vi "Value Pair Page.vi"() -> ()   [LabVIEW 2020, in "3D Plot.lvclass"]
uses:
  <vilib>/Math Plots/3D Math Plots/3D Plot/3D Plot/3D Plot.lvclass
  <vilib>/Math Plots/3D Math Plots/3D Plot/3D Plot/Typedef/Value Pair Property.ctl
  <vilib>/Math Plots/3D Math Plots/3D Plot/3D Plot/Typedef/Value Pair Cluster.ctl
  <vilib>/Math Plots/3D Math Plots/3D Plot/3D Plot/Typedef/Dialog State.ctl
  <vilib>/Math Plots/3D Math Plots/3D Plot/3D Plot/Typedef/Temp Scene State.ctl
  <vilib>/Math Plots/3D Math Plots/3D Plot/3D Plot/Typedef/Temp Scene Property Action.ctl
panel:
  in  "Move Down":bool caption="Move down"
  in  "Move Up":bool caption="Move up"
  in  "Delete":bool
  in  "New":bool
  in  "Active Axis":u16(ring) caption="Active axis" items=["X Axis", "Y Axis", "Z Axis"]
  in  "Label Mode":u16(ring) caption="Label mode" items=["Name", "Value", "None "]
  in  "Show Tick":bool caption="Show tick"
  in  "Show Grid":bool caption="Show grid"
  in  "Value":sgl
  in  "Name":string
  in  "Value Pair List":i32(listbox) caption="Value pair list"
  out "Value Pair Property Out":T1
  in  "Value Pair Property In":T1
  in  "Event Registration":refnum<event-registration>
  # "Value Pair"
  # "Display Style"
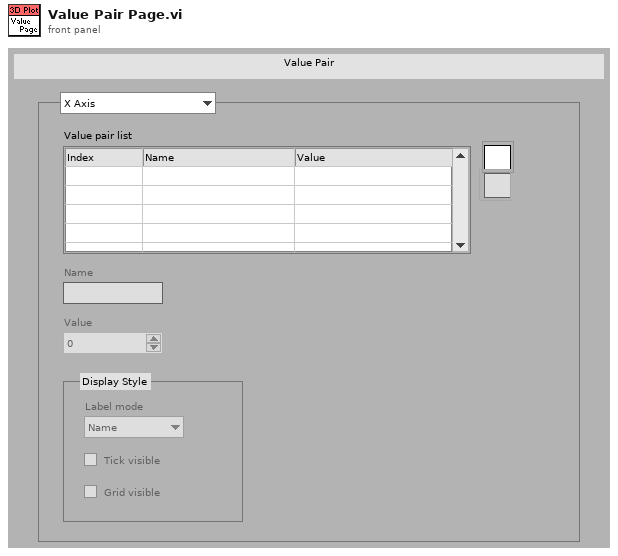
[diagram p1: front panel]
types:
  T1 = typedef "3D Plot.lvclass/Value Pair Property.ctl" = T2[]
  T2 = typedef "3D Plot.lvclass/Value Pair Cluster.ctl" = cluster{"Value Pair Array":cluster{"Value":sgl, "Name":string}[], "Show Tick":bool, "Show Grid":bool, " Label Mode":enum16{"Name", "Value", "None"}}
  T3 = typedef "3D Plot.lvclass/Dialog State.ctl" = enum16{"Initialize", "Read Porperty", "Write Property", "Idle", "Exit"}
  T4 = typedef "3D Plot.lvclass/Temp Scene Property Action.ctl" = enum16{"Graph Property", "Light Property", "Axis Property", "Value Pair Property", "Format Property", "Cursor Property", "Plot Specific Property"}
  T5 = typedef "3D Plot.lvclass/Temp Scene State.ctl" = enum16{"Create", "Update Scene", "Get Plot Representation", "Destory"}
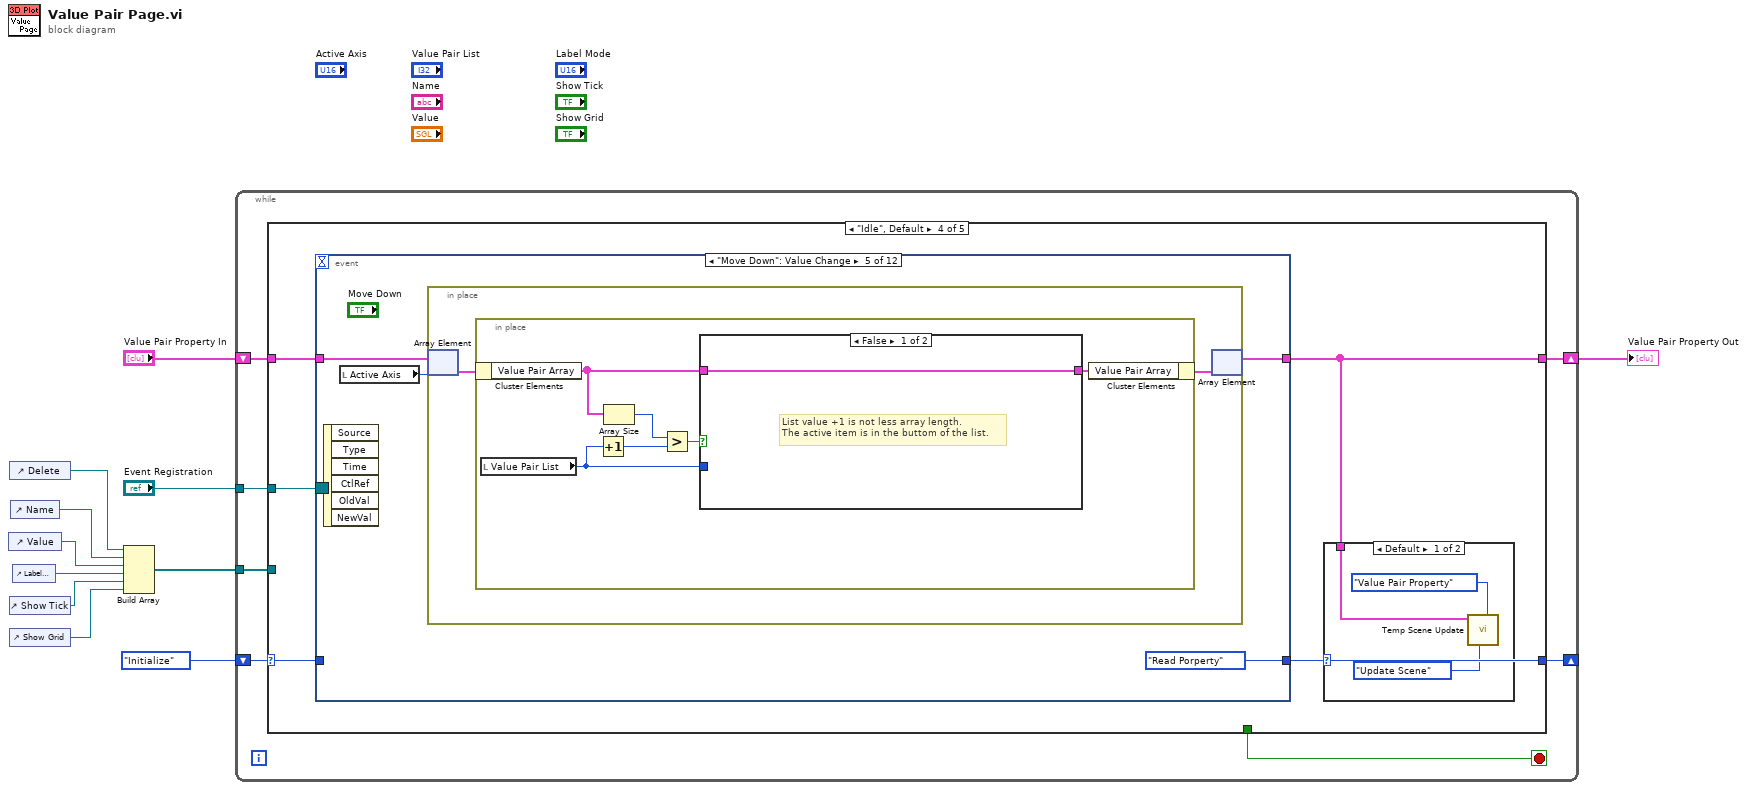
[diagram p0: block diagram]
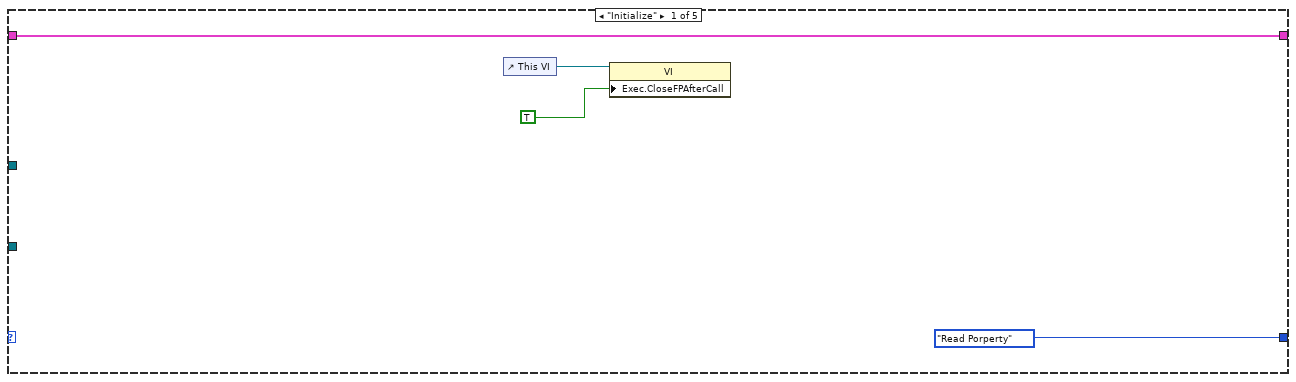
[diagram p2: hidden frame]
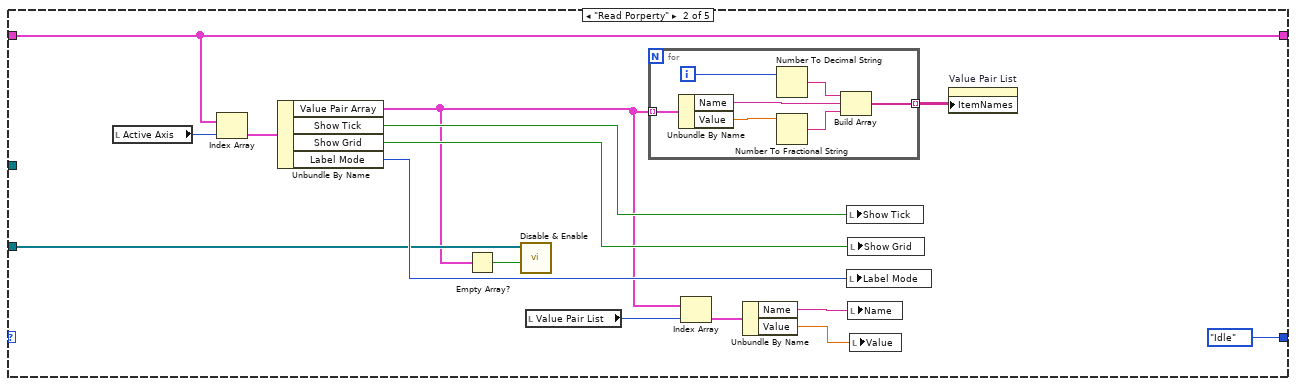
[diagram p3: hidden frame]
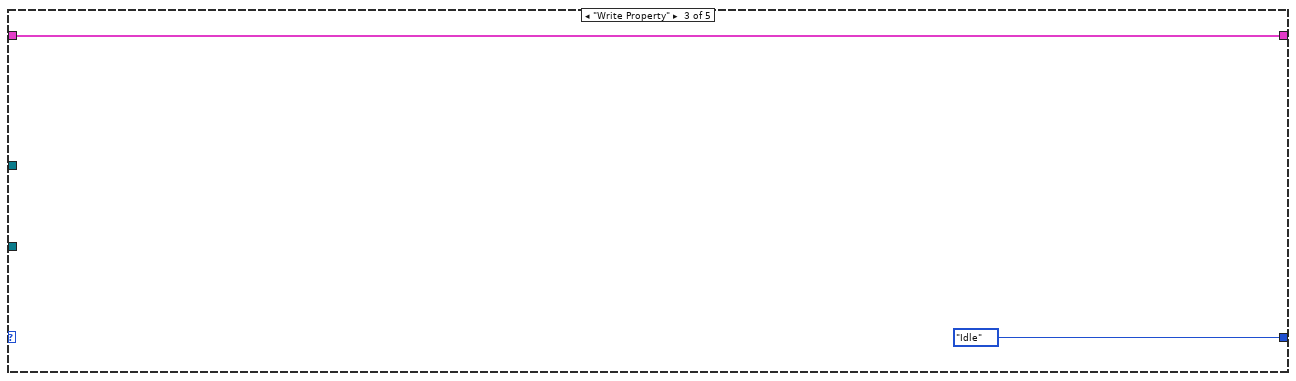
[diagram p4: hidden frame]
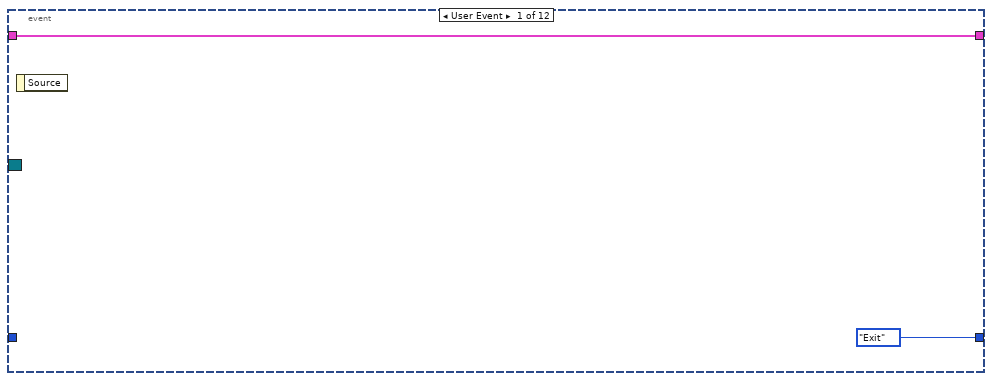
[diagram p6: hidden frame]
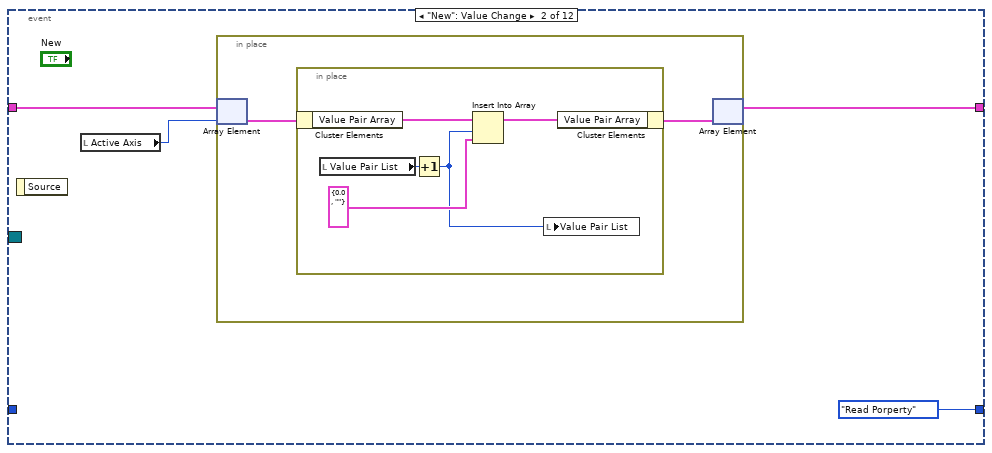
[diagram p7: hidden frame]
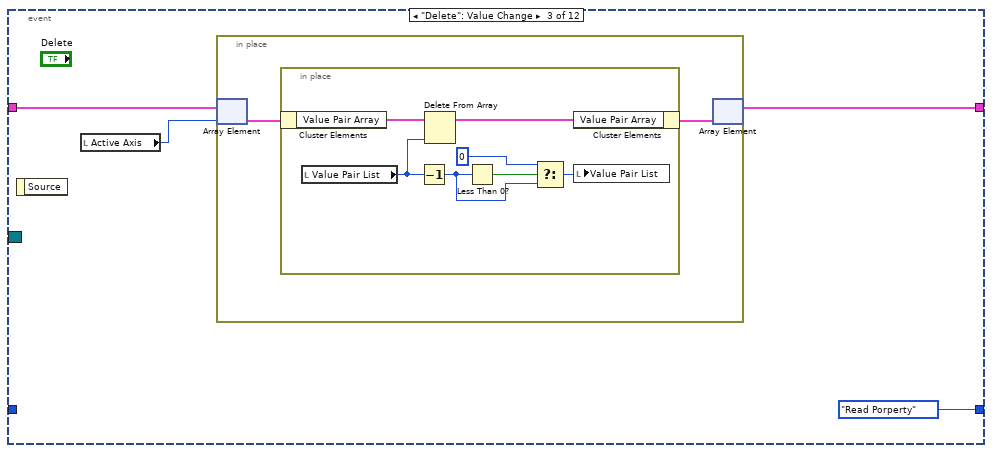
[diagram p8: hidden frame]
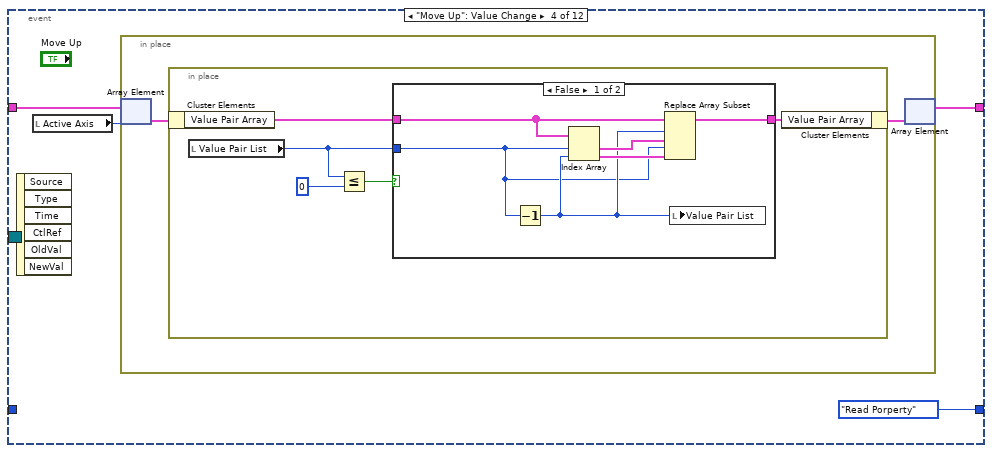
[diagram p9: hidden frame]
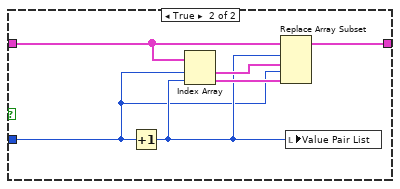
[diagram p11: hidden frame]
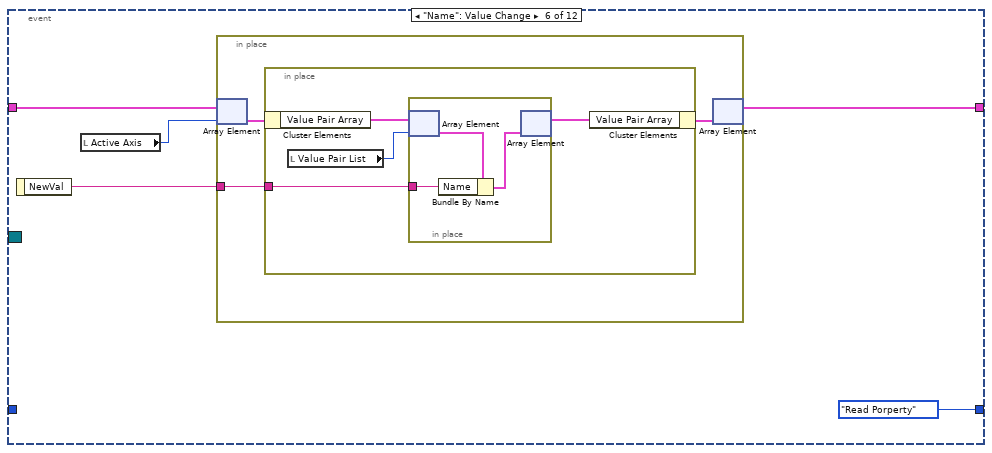
[diagram p12: hidden frame]
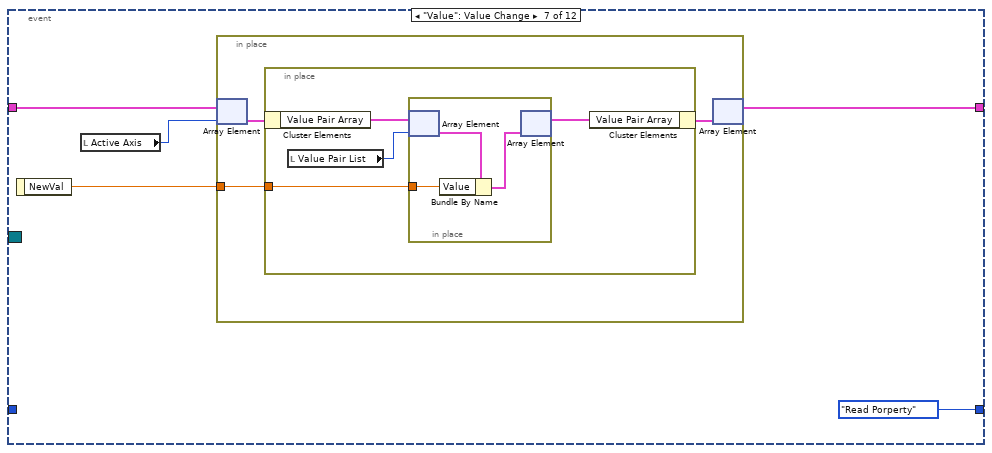
[diagram p13: hidden frame]
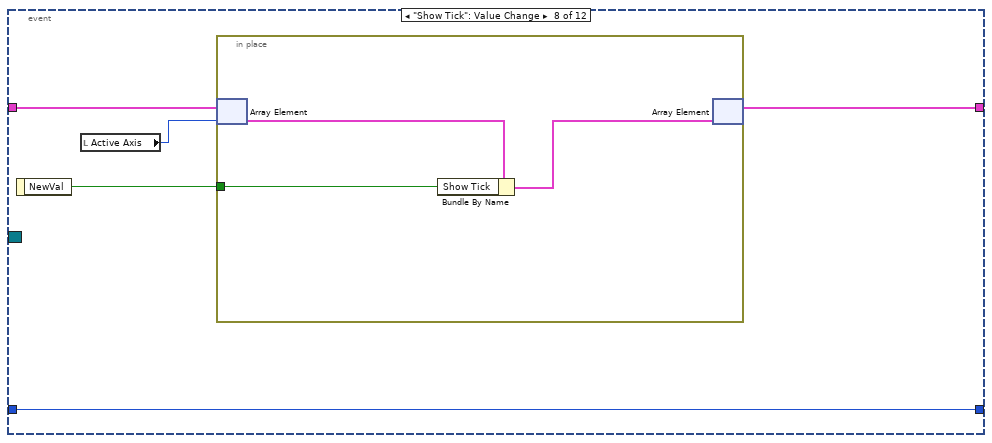
[diagram p14: hidden frame]
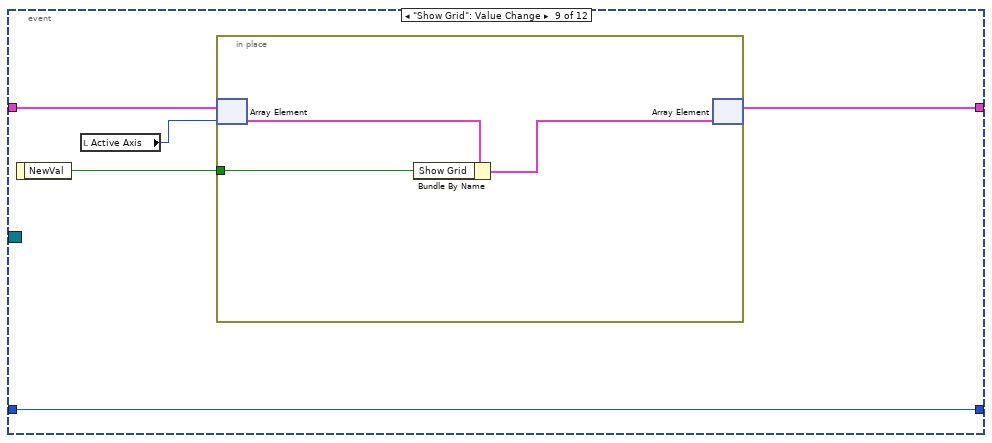
[diagram p15: hidden frame]
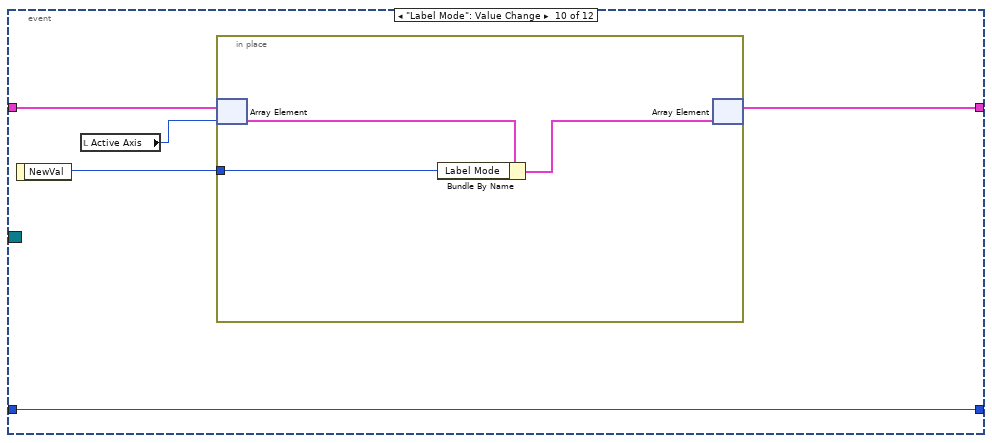
[diagram p16: hidden frame]
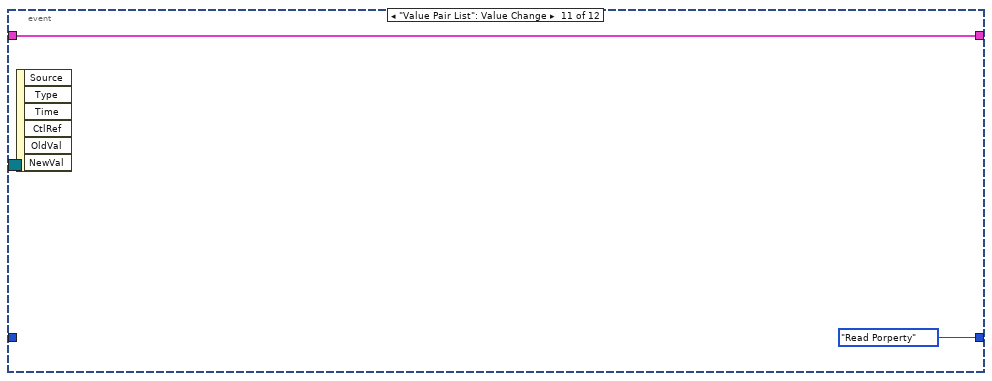
[diagram p17: hidden frame]
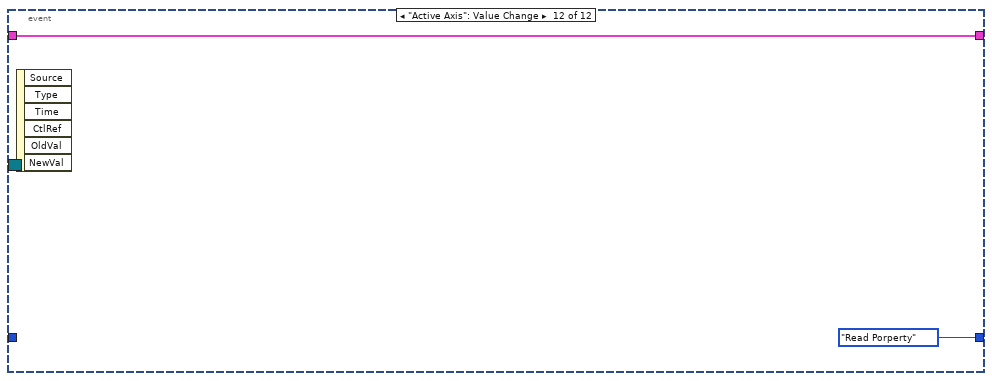
[diagram p18: hidden frame]
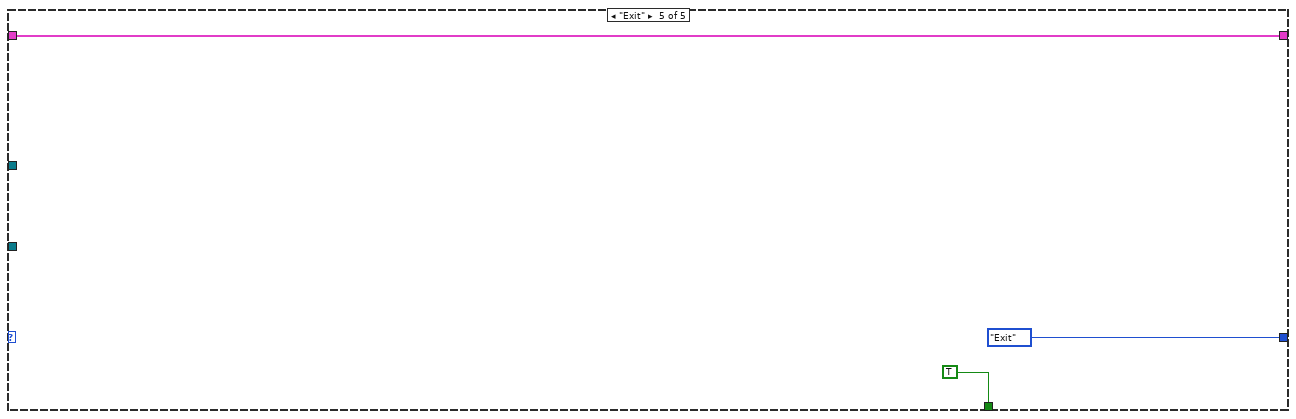
[diagram p19: hidden frame]
diagram:
  n1 = control-ref of="Value"() -> (w6:refnum<vi>)
  n2 = control-ref of="Delete"() -> (w1:refnum<vi>)
  n3 = control-ref of="Show Tick"() -> (w4:refnum<vi>)
  n4 = control-ref of="Show Grid"() -> (w3:refnum<vi>)
  n5 = control-ref of="Name"() -> (w7:refnum<vi>)
  n6 = control-ref of="Label Mode"() -> (w5:refnum<vi>)
  n7 = Build Array(w1, w7, w6, w5, w4, w3) -> (w2:refnum<vi>[])
  n8 = while {
    shift-right: [w17] -> w8
    shift-left: "Value Pair Property In" -> [w18]
    shift-right: [w13] -> _
    shift-left: Dialog_State."Initialize" -> [w16]
    tunnel: "Event Registration" -> [w14]
    tunnel: w2 -> [w12]
    stop <- w15 stop-if-true
    n9 = case shown="\"Idle\", Default" w16 {
      selector: w16 -> [_ _ _ w49 _]
      tunnel: w18 -> [w21 w25 w45 w51 w176]
      tunnel: [w21 w25 w45 w48 w176] -> w17
      tunnel: [Dialog_State."Read Porperty" Dialog_State."Idle" Dialog_State."Idle" w47 Dialog_State."Exit"] -> w13
      tunnel: [_ _ _ _ TRUE] -> w15
      tunnel: w14 -> [_ _ _ w50 _]
      tunnel: w12 -> [_ w26 _ _ _]
      frame "Initialize" {
        n10 = control-ref of="This VI"() -> (w20:refnum<vi>)
        n11 = property class="VI"(reference=w20, "Exec.CloseFPAfterCall"=TRUE ("Execution:Close After Call")) -> ()  [unwired: 1 in, 2 out]
      }
      frame "Read Porperty" {
        n12 = local read "Active Axis"() -> (w36:u16)
        n13 = Index Array(array=w25, index=w36) -> (element=w35:T2)
        n14 = Unbundle By Name(w35) -> ("Value Pair Array"=w23:cluster{"Value":sgl, "Name":string}[], "Show Tick"=w33:bool, "Show Grid"=w32:bool, "Label Mode"=w34:enum16{"Name", "Value", "None"})
        n15 = Empty Array?(array=w23) -> (empty?=w24:bool)
        n16 = call <vilib>:"Disable & Enable.vi"("Disabled?"=w24, "Control Ref Array"=w26) -> ()  [unwired: 1 in, 9 out]
        n17 = local read "Value Pair List"() -> (w27:i32)
        n18 = for {
          tunnel: w23 -> [w44] mode=indexing
          tunnel: [w39] -> w28 mode=indexing
          i -> [w38]
          n19 = Unbundle By Name(w44) -> ("Name"=w41:string, "Value"=w43:sgl)
          n20 = Number To Decimal String(number=w38) -> (decimal integer string=w42:string)  [unwired: 1 out]
          n21 = Number To Fractional String(number=w43) -> (F-format string=w40:string)  [unwired: 3 out]
          n22 = Build Array(w42, w41, w40) -> (w39:string[])
        }
        n23 = Index Array(array=w23, index=w27) -> (element=w31:cluster{"Value":sgl, "Name":string})
        n24 = Unbundle By Name(w31) -> ("Name"=w30:string, "Value"=w29:sgl)
        n25 = local write "Show Tick"(w33) -> ()
        n26 = local write "Label Mode"(w34) -> ()
        n27 = local write "Show Grid"(w32) -> ()
        n28 = local write "Name"(w30) -> ()
        n29 = local write "Value"(w29) -> ()
        n30 = property on="Value Pair List" class="MCListbox (strict)"("ItemNames"=w28) -> ()  [unwired: 2 in, 2 out]
      }
      frame "Write Property" {
      }
      frame "Idle", Default {
        n31 = event shown="[4] \"Move Down\": Value Change" {
          selector: w50 -> [_ _ _ _ _ _ _ _ _ _ _ _]
          dyn-events: _ -> [_ _ _ _ _ _ _ _ _ _ _ _]
          timeout: _ -> [_ _ _ _ _ _ _ _ _ _ _ _]
          tunnel: w51 -> [w56 w60 w71 w84 w102 w122 w136 w152 w160 w168 w173 w175]
          tunnel: [w56 w59 w70 w82 w100 w121 w135 w151 w159 w166 w173 w175] -> w48
          tunnel: [Dialog_State."Exit" Dialog_State."Read Porperty" Dialog_State."Read Porperty" Dialog_State."Read Porperty" Dialog_State."Read Porperty" Dialog_State."Read Porperty" Dialog_State."Read Porperty" w148 w156 w164 Dialog_State."Read Porperty" Dialog_State."Read Porperty"] -> w47
          tunnel: w49 -> [_ _ _ _ _ _ _ w148 w156 w164 _ _]
          event User Event {
            n32 = event-data() -> ()  [unwired: 2 out]
          }
          event "New": Value Change {
            n33 = event-data() -> ()  [unwired: 2 out]
            n34 = local read "Active Axis"() -> (w57:u16)
            n35 = in-place {
              n36 = in-place-array #1(w60, w57) -> (w62:T2)
              n37 = in-place {
                n38 = in-place-cluster #2(w62) -> ("Value Pair Array"=w67:cluster{"Value":sgl, "Name":string}[])
                n39 = local read "Value Pair List"() -> (w64:i32)
                n40 = Increment(x=w64) -> (x+1=w63:i32)
                n41 = Insert Into Array(array=w67, index=w63, new element=cluster{"Value":dbl, "Name":string} {"Value"=0.0, "Name"=""} ("new element/subarray")) -> (w66:cluster{"Value":sgl, "Name":string}[])
                n42 = local write "Value Pair List"(w63) -> ()
                n43 = in-place-cluster #2("Value Pair Array"=w66) -> (w61:T2)
              }
              n44 = in-place-array #1(w61) -> (w59:T1)  [unwired: 1 out]
            }
          }
          event "Delete": Value Change {
            n45 = event-data() -> ()  [unwired: 2 out]
            n46 = local read "Active Axis"() -> (w68:u16)
            n47 = in-place {
              n48 = in-place-array #3(w71, w68) -> (w73:T2)
              n49 = in-place {
                n50 = in-place-cluster #4(w73) -> ("Value Pair Array"=w80:cluster{"Value":sgl, "Name":string}[])
                n51 = local read "Value Pair List"() -> (w78:i32)
                n52 = Decrement(x=w78) -> (x-1=w75:i32)
                n53 = Delete From Array(array=w80, index=w78) -> (array with subset deleted=w79:cluster{"Value":sgl, "Name":string}[])  [unwired: 1 in, 1 out]
                n54 = Less Than 0?(x=w75) -> (x < 0?=w77:bool)
                n55 = Select(t=0, s=w77, f=w75) -> (s? t:f=w74:i32)
                n56 = in-place-cluster #4("Value Pair Array"=w79) -> (w72:T2)
                n57 = local write "Value Pair List"(w74) -> ()
              }
              n58 = in-place-array #3(w72) -> (w70:T1)  [unwired: 1 out]
            }
          }
          event "Move Up": Value Change {
            n59 = event-data() -> ()  [unwired: 7 out]
            n60 = local read "Active Axis"() -> (w83:u16)
            n61 = in-place {
              n62 = in-place-array #5(w84, w83) -> (w86:T2)
              n63 = in-place {
                n64 = in-place-cluster #6(w86) -> ("Value Pair Array"=w91:cluster{"Value":sgl, "Name":string}[])
                n65 = local read "Value Pair List"() -> (w87:i32)
                n66 = Less Or Equal?(x=w87, y=0) -> (x <= y?=w88:bool)
                n67 = case shown="False" w88 {
                  tunnel: w91 -> [w97 w98]
                  tunnel: [w96 w98] -> w90
                  tunnel: w87 -> [w92 _]
                  frame False {
                    n68 = Decrement(x=w92) -> (x-1=w93:i32)
                    n69 = Index Array(array=w97, index #1=w92, index #2=w93) -> (element #1=w95:cluster{"Value":sgl, "Name":string}, element #2=w94:cluster{"Value":sgl, "Name":string})
                    n70 = Replace Array Subset(array=w97, new element #1=w95, index #1=w93, new element #2=w94, index #2=w92) -> (w96:cluster{"Value":sgl, "Name":string}[])
                    n71 = local write "Value Pair List"(w93) -> ()
                  }
                  frame True {
                    # "List value is less or equal to 0.\nThe active item is in the top of the list."
                  }
                }
                n72 = in-place-cluster #6("Value Pair Array"=w90) -> (w85:T2)
              }
              n73 = in-place-array #5(w85) -> (w82:T1)  [unwired: 1 out]
            }
          }
          event "Move Down": Value Change {
            n74 = event-data() -> ()  [unwired: 7 out]
            n75 = local read "Active Axis"() -> (w101:u16)
            n76 = in-place {
              n77 = in-place-array #7(w102, w101) -> (w103:T2)
              n78 = in-place {
                n79 = in-place-cluster #8(w103) -> ("Value Pair Array"=w109:cluster{"Value":sgl, "Name":string}[])
                n80 = local read "Value Pair List"() -> (w105:i32)
                n81 = Increment(x=w105) -> (x+1=w107:i32)
                n82 = Array Size(array=w109) -> (size(s)=w108:i32)
                n83 = Greater?(x=w108, y=w107) -> (0:w106:bool)
                n84 = case shown="False" w106 {
                  tunnel: w109 -> [w111 w117]
                  tunnel: [w111 w116] -> w110
                  tunnel: w105 -> [_ w112]
                  frame False {
                    # "List value +1 is not less array length.\nThe active item is in the buttom of the list."
                  }
                  frame True {
                    n85 = Increment(x=w112) -> (x+1=w113:i32)
                    n86 = Index Array(array=w117, index #1=w112, index #2=w113) -> (element #1=w115:cluster{"Value":sgl, "Name":string}, element #2=w114:cluster{"Value":sgl, "Name":string})
                    n87 = Replace Array Subset(array=w117, new element #1=w115, index #1=w113, new element #2=w114, index #2=w112) -> (w116:cluster{"Value":sgl, "Name":string}[])
                    n88 = local write "Value Pair List"(w113) -> ()
                  }
                }
                n89 = in-place-cluster #8("Value Pair Array"=w110) -> (w104:T2)
              }
              n90 = in-place-array #7(w104) -> (w100:T1)  [unwired: 1 out]
            }
          }
          event "Name": Value Change {
            n91 = event-data() -> ("NewVal"=w119:string)  [unwired: 1 out]
            n92 = local read "Active Axis"() -> (w120:u16)
            n93 = in-place {
              in-place-border: w119 -> [w123]
              n94 = in-place-array #9(w122, w120) -> (w125:T2)
              n95 = in-place {
                in-place-border: w123 -> [w126]
                n96 = in-place-cluster #10(w125) -> ("Value Pair Array"=w129:cluster{"Value":sgl, "Name":string}[])
                n97 = local read "Value Pair List"() -> (w127:i32)
                n98 = in-place {
                  in-place-border: w126 -> [w130]
                  n99 = in-place-array #11(w129, w127) -> (w132:cluster{"Value":sgl, "Name":string})
                  n100 = Bundle By Name(cluster=w132, "Name"=w130) -> (w131:cluster{"Value":sgl, "Name":string})
                  n101 = in-place-array #11(w131) -> (w128:cluster{"Value":sgl, "Name":string}[])  [unwired: 1 out]
                }
                n102 = in-place-cluster #10("Value Pair Array"=w128) -> (w124:T2)
              }
              n103 = in-place-array #9(w124) -> (w121:T1)  [unwired: 1 out]
            }
          }
          event "Value": Value Change {
            n104 = event-data() -> ("NewVal"=w134:sgl)  [unwired: 1 out]
            n105 = local read "Active Axis"() -> (w137:u16)
            n106 = in-place {
              in-place-border: w134 -> [w138]
              n107 = in-place-array #12(w136, w137) -> (w140:T2)
              n108 = in-place {
                in-place-border: w138 -> [w141]
                n109 = in-place-cluster #13(w140) -> ("Value Pair Array"=w144:cluster{"Value":sgl, "Name":string}[])
                n110 = local read "Value Pair List"() -> (w142:i32)
                n111 = in-place {
                  in-place-border: w141 -> [w145]
                  n112 = in-place-array #14(w144, w142) -> (w147:cluster{"Value":sgl, "Name":string})
                  n113 = Bundle By Name(cluster=w147, "Value"=w145) -> (w146:cluster{"Value":sgl, "Name":string})
                  n114 = in-place-array #14(w146) -> (w143:cluster{"Value":sgl, "Name":string}[])  [unwired: 1 out]
                }
                n115 = in-place-cluster #13("Value Pair Array"=w143) -> (w139:T2)
              }
              n116 = in-place-array #12(w139) -> (w135:T1)  [unwired: 1 out]
            }
          }
          event "Show Tick": Value Change {
            n117 = event-data() -> ("NewVal"=w149:bool)  [unwired: 1 out]
            n118 = local read "Active Axis"() -> (w150:u16)
            n119 = in-place {
              in-place-border: w149 -> [w153]
              n120 = in-place-array #15(w152, w150) -> (w155:T2)
              n121 = Bundle By Name(cluster=w155, "Show Tick"=w153) -> (w154:T2)
              n122 = in-place-array #15(w154) -> (w151:T1)  [unwired: 1 out]
            }
          }
          event "Show Grid": Value Change {
            n123 = event-data() -> ("NewVal"=w157:bool)  [unwired: 1 out]
            n124 = local read "Active Axis"() -> (w158:u16)
            n125 = in-place {
              in-place-border: w157 -> [w162]
              n126 = in-place-array #16(w160, w158) -> (w163:T2)
              n127 = Bundle By Name(cluster=w163, "Show Grid"=w162) -> (w161:T2)
              n128 = in-place-array #16(w161) -> (w159:T1)  [unwired: 1 out]
            }
          }
          event "Label Mode": Value Change {
            n129 = event-data() -> ("NewVal"=w165:u16)  [unwired: 1 out]
            n130 = local read "Active Axis"() -> (w167:u16)
            n131 = in-place {
              in-place-border: w165 -> [w169]
              n132 = in-place-array #17(w168, w167) -> (w171:T2)
              n133 = Bundle By Name(cluster=w171, "Label Mode"=w169) -> (w170:T2)
              n134 = in-place-array #17(w170) -> (w166:T1)  [unwired: 1 out]
            }
          }
          event "Value Pair List": Value Change {
            n135 = event-data() -> ()  [unwired: 7 out]
          }
          event "Active Axis": Value Change {
            n136 = event-data() -> ()  [unwired: 7 out]
          }
        }
        n137 = case shown="Default" w47 {
          tunnel: w48 -> [w52 _]
          frame Default {
            n138 = call <vilib>:"Temp Scene Update.vi"("Property Name"=Temp_Scene_Property_Action."Value Pair Property", "State"=Temp_Scene_State."Update Scene", "Property In"=w52) -> ()  [unwired: 3 in, 6 out]
          }
          frame "Exit" {
          }
        }
      }
      frame "Exit" {
      }
    }
  }
  "Value Pair Property Out" <- w8
